vi "FTW-TestExecutive-Core_OnStepChange.vi"(0 "FTW-Scripter-Core In":refnum<class "FTW-TestExecutive-Core.lvclass">, 11 "error in":errorcluster) -> (4 "FTW-Scripter-Core Out":refnum<class "FTW-TestExecutive-Core.lvclass">, 15 "error out":errorcluster)   [LabVIEW 2015, in "FTW-TestExecutive-Core.lvclass"]
uses:
  FTW-TestExecutive-Core.lvclass
  FTW-TestExecutive-Core.lvclass/FTW-TestExecutive-Core.ctl
  source/actor/Instance-Extended/FTW-ActorExtended.lvclass
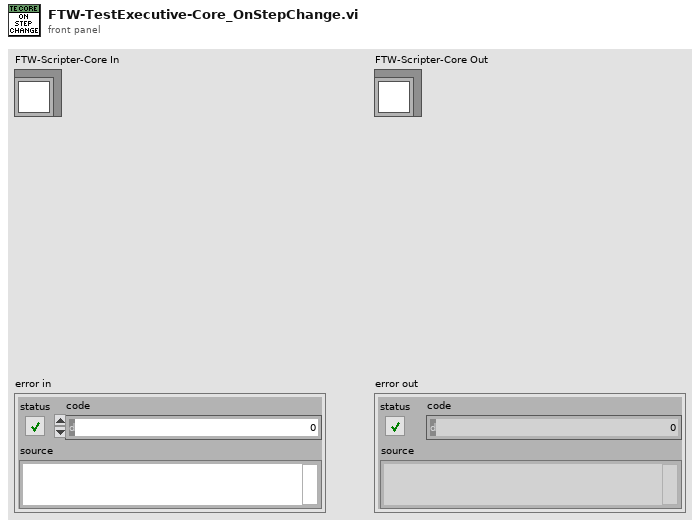
[diagram p1: front panel]
types:
  T1 = typedef "FTW-TestExecutive_Step.ctl" = cluster{"Name":string, "Type":string, "Path":string, "Config":string, "Elapsed Time":dbl, "Passed":bool}
  T2 = cluster{"Sequence":T1[], "Current Step Index":i32}
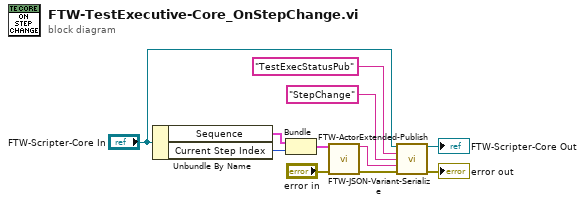
[diagram p0: block diagram]
diagram:
  n1 = Unbundle By Name("FTW-Scripter-Core In") -> ("Sequence"=w2:T1[], "Current Step Index"=w1:i32)
  n2 = Bundle("Sequence"=w2, "Current Step Index"=w1) -> (w3:T2)  [unwired: 1 in]
  n3 = call "FTW-JSON-Variant-Serialize.vi"("Variant"=w3, "error in"="error in") -> ("JSON String"=w4:string, "error out"=w5:errorcluster)  [unwired: 12 in]
  n4 = call "FTW-ActorExtended-Publish.vi"("FTW-ActorExtended In"="FTW-Scripter-Core In", "Publisher Name"="TestExecStatusPub", "Message Header"="StepChange", "Message Body"=w4, "error in"=w5) -> ("FTW-ActorExtended Out"=→"FTW-Scripter-Core Out":refnum<class "FTW-TestExecutive-Core.lvclass">, "error out"=→"error out":errorcluster)  [unwired: 9 in]
